vi "Main.vi"(10 "SerialPort":u8=1, 11 "Module Admin":refnum<class "Delacor_lib_QMH_Module Admin.lvclass">) -> ()   [LabVIEW 2020, in "SMC100.lvlib"]
doc: "This template is based off of the Queued Message Handler design pattern and the Queued Message Handler project template that ships with LabVIEW.\n\nThe main difference is that the queue is private to this module and communication between modules is performed via Broadcast and Request events.\n\nRequest events are wrapped in public API methods and are handled in the Event Handling Loop (EHL) of this VI. Any module can register for Broadcast events sent by this module. The EHL generates messages based on user interface actions.\n\nThe Message Handling Loop (MHL) processes messages generated by the EHL, or by other messages. The messages are string values, so new messages can be added easily to the Message Cases case structure in the MHL. Each message cluster can also provide an optional value for Message Data, which is a variant that can be converted to whatever message-specific data is required.\n_____\nBased on Delacor QMH Project Template 5.0.0.82."
uses:
  SMC100.lvlib
  <vilib>/Delacor/Delacor QMH/Libraries/Module Admin_class/Delacor_lib_QMH_Module Admin.lvclass
  Module Data--cluster.ctl
  Stop Argument--cluster.ctl
  <vilib>/Delacor/Delacor QMH/Libraries/Message Queue_class/Delacor_lib_QMH_Message Queue.lvclass/Delacor_lib_QMH_Message Queue.ctl
  <vilib>/Delacor/Delacor QMH/Libraries/Module Admin_class/Delacor_lib_QMH_Module Admin.lvclass/Delacor_lib_QMH_Module Admin.ctl
  Get Abs Position Argument--cluster.ctl
  Get Abs Position (Reply Payload)--cluster.ctl
  Set Abs Position Argument--cluster.ctl
  Move Home Argument--cluster.ctl
  <vilib>/Utility/miscctls.llb/LVPointTypeDef.ctl
  <vilib>/Delacor/Delacor QMH/Libraries/Message Queue_class/Delacor_lib_QMH_Enqueue Message (Single).vi
  <vilib>/Delacor/Delacor QMH/Libraries/Module Admin_class/Delacor_lib_QMH_Get External Launch.vi
  SMC100-Controller-Drivers/SMC100.llb/enter / leave disable state.vi
  <vilib>/Utility/error.llb/Error Cluster From Error Code.vi
  <vilib>/ErrorRing/Error Ring.xnode
  <vilib>/Delacor/Delacor QMH/Libraries/Message Queue_class/Delacor_lib_QMH_Message Queue.lvclass
panel:
  in  "Target Position":dbl format="%_4g"
  out "Absolute Position":dbl format="%_4g"
  out "Controller's state":string
  out "Controller's error":string
  out "error out":errorcluster
  out "Status":string
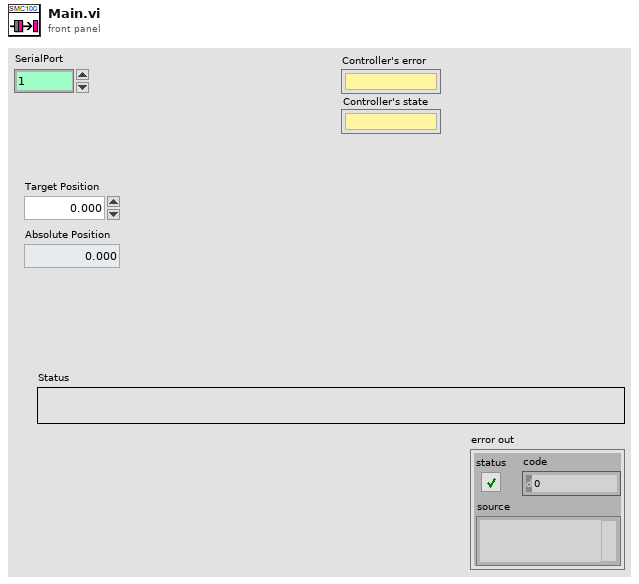
[diagram p1: front panel]
types:
  T1 = typedef "SMC100.lvlib/Request Events--cluster.ctl" = cluster{"Stop Module":refnum<user-event>, "Show Panel":refnum<user-event>, "Hide Panel":refnum<user-event>, "Get Module Execution Status":refnum<user-event>, "Show Diagram":refnum<user-event>, "Get Abs Position":refnum<user-event>, "Set Abs Position":refnum<user-event>, "Move Home":refnum<user-event>}
  T2 = typedef "SMC100.lvlib/Module Data--cluster.ctl" = cluster{"Status":string, "Visa Handle":refnum<visa-resource-name>}
  T3 = enum32{"invalid lock state", "Not Locked", "Locked (No Password)", "Password-protected"}
  T4 = typedef "SMC100.lvlib/Stop Argument--cluster.ctl" = cluster{"Origin":string, "Exit via Stop Module Req?":bool, "Wait for Module to stop?":bool}
  T5 = typedef "SMC100.lvlib/Get Abs Position Argument--cluster.ctl" = cluster{"Wait Notifier":refnum<notifier>, "wait for reply":bool}
  T6 = typedef "SMC100.lvlib/Set Abs Position Argument--cluster.ctl" = cluster{"Abolute Position":dbl}
  T7 = typedef "SMC100.lvlib/Move Home Argument--cluster.ctl" = cluster{"Boolean":bool}
  T8 = typedef "LVPointTypeDef.ctl" = cluster{"Horizontal":i16, "Vertical":i16}
  T9 = enum32{"Invalid", "Standard", "Closed", "Hidden", "Minimized", "Maximized"}
  T10 = typedef "SMC100.lvlib/Get Abs Position (Reply Payload)--cluster.ctl" = cluster{"Absolute Position":dbl, "Get Abs Position_error":errorcluster}
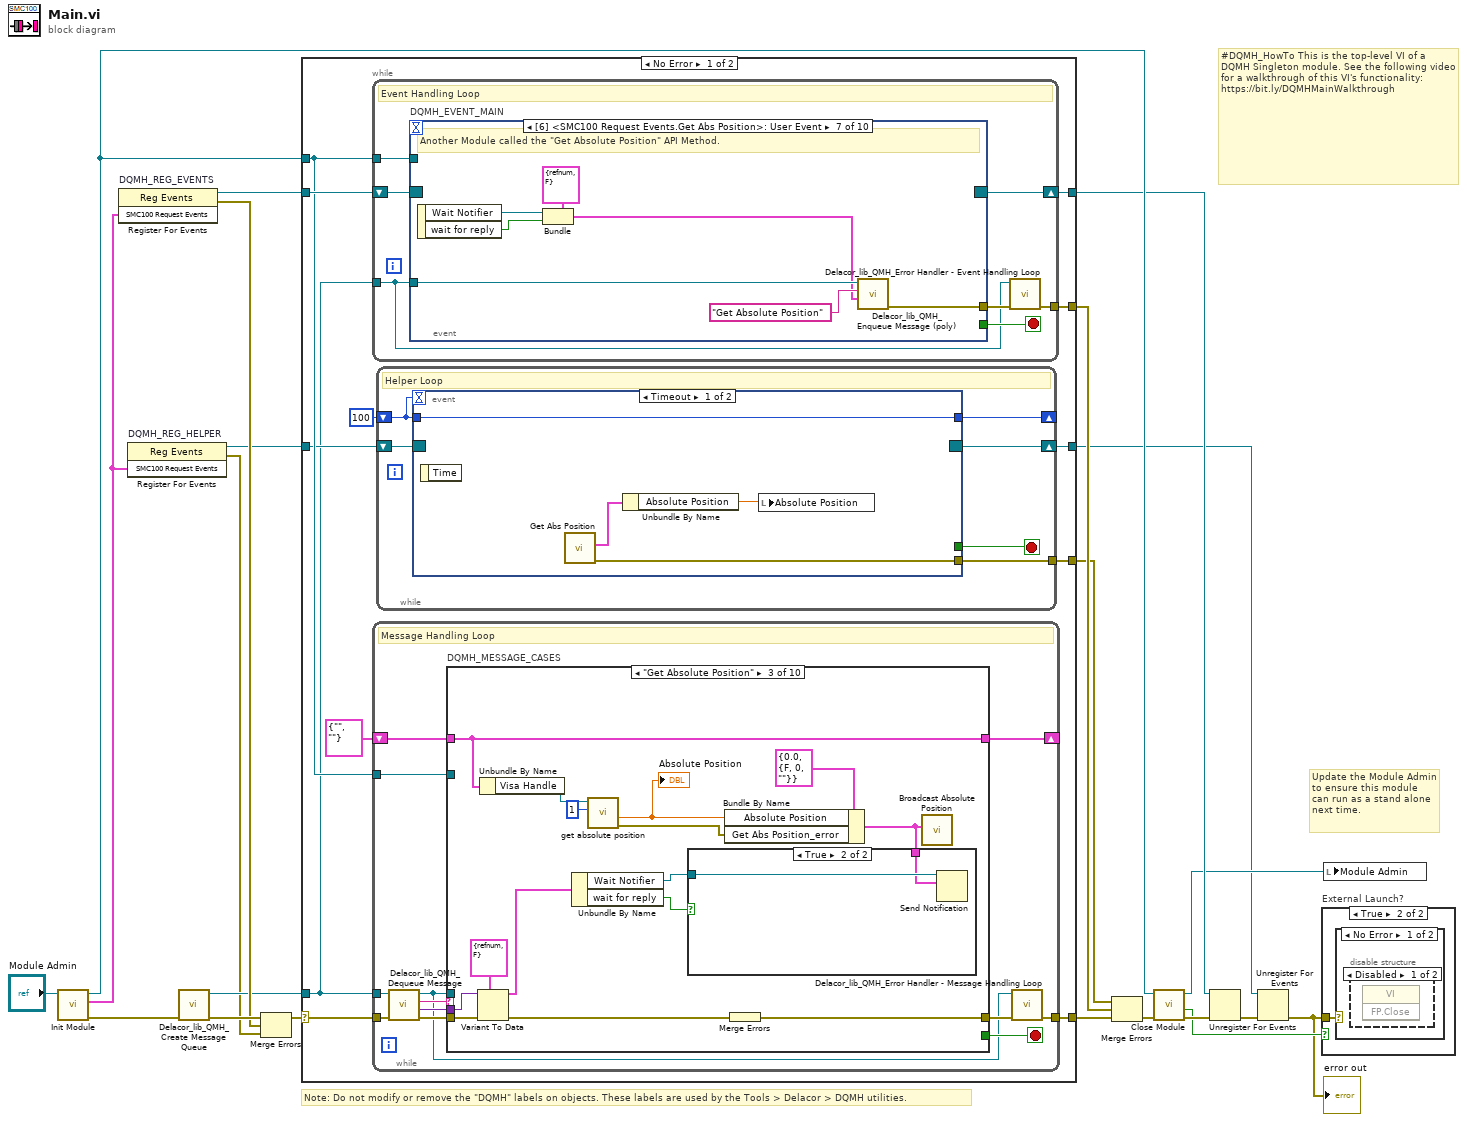
[diagram p0: block diagram]
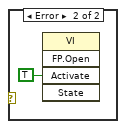
[diagram p4: hidden frame]
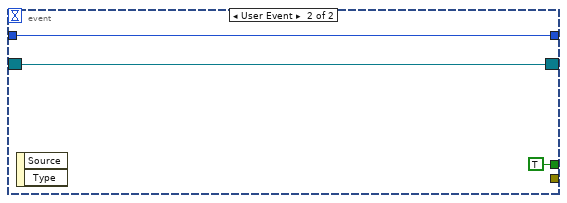
[diagram p5: hidden frame]
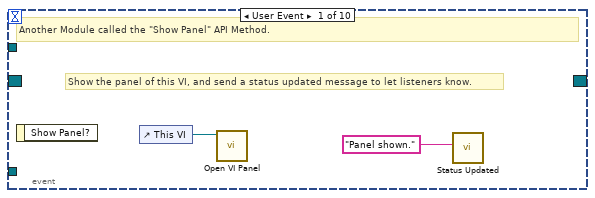
[diagram p6: hidden frame]
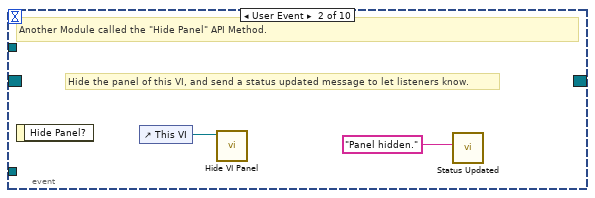
[diagram p7: hidden frame]
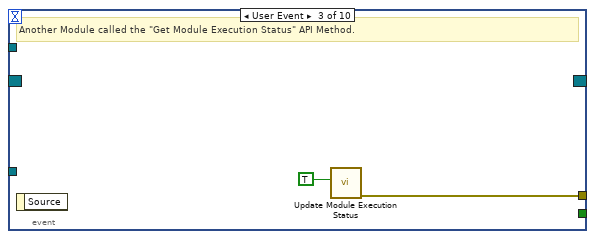
[diagram p8: hidden frame]
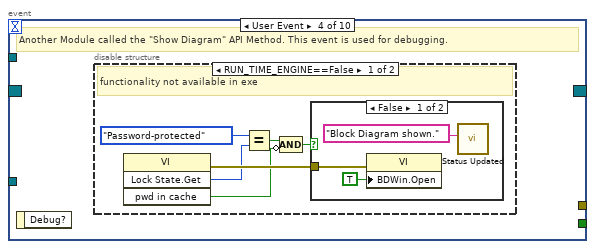
[diagram p9: hidden frame]
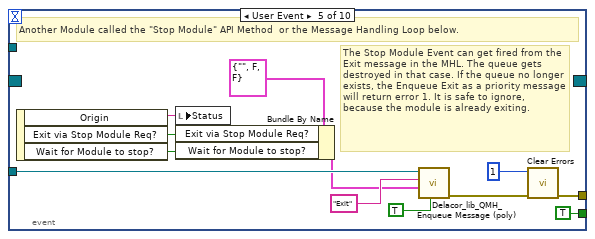
[diagram p12: hidden frame]
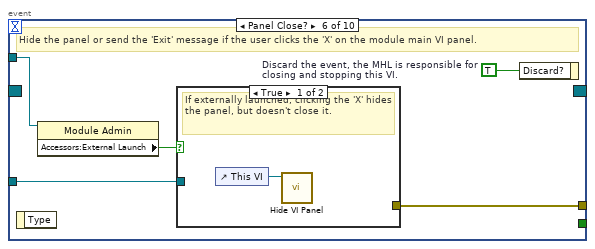
[diagram p13: hidden frame]
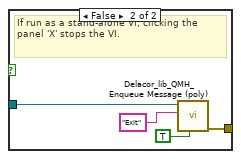
[diagram p14: hidden frame]
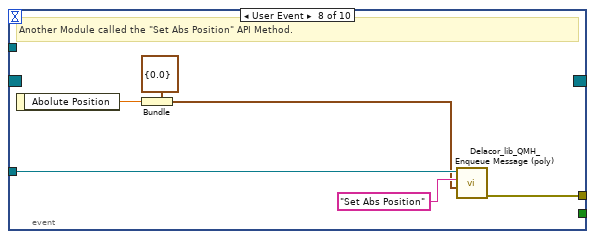
[diagram p15: hidden frame]
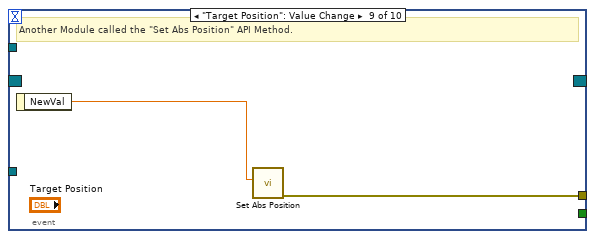
[diagram p16: hidden frame]
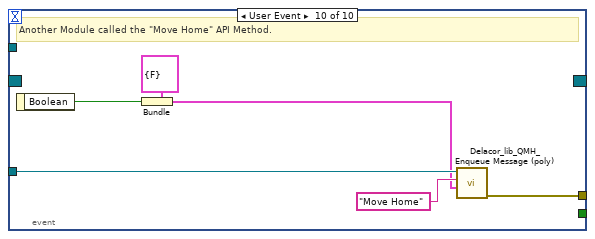
[diagram p17: hidden frame]
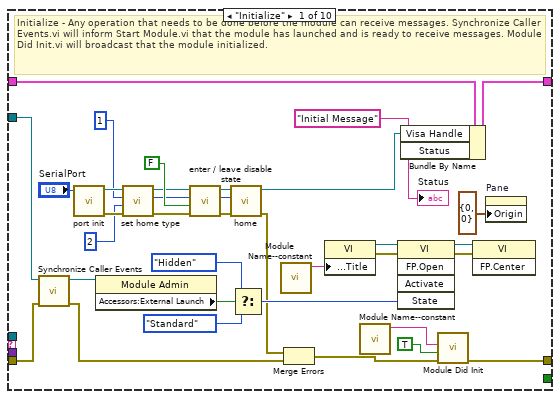
[diagram p18: hidden frame]
diagram:
  # "#DQMH_HowTo This is the top-level VI of a DQMH Singleton module. See the following video for a walkthrough of this VI's functionality: https://bit.ly/DQMHMainWalkthrough"
  # "Note: Do not modify or remove the \"DQMH\" labels on objects. These labels are used by the Tools > Delacor > DQMH utilities."
  # "Update the Module Admin to ensure this module can run as a stand alone next time."
  n1 = call "Init Module.vi"("Singleton Module Admin in"="Module Admin") -> ("error out"=w21:errorcluster, "SMC100 Request Events"=w4:T1, "Singleton Module Admin out"=w13:refnum<class "Delacor_lib_QMH_Module Admin.lvclass">)  [unwired: 8 in]
  n2 = register-events "DQMH_REG_EVENTS"(w4) -> (reference out=w11:refnum<event-registration>, error out=w14:errorcluster)  [unwired: 2 in]
  n3 = register-events "DQMH_REG_HELPER"(w4) -> (reference out=w6:refnum<event-registration>, error out=w5:errorcluster)  [unwired: 2 in]
  n4 = call <vilib>:"Delacor_lib_QMH_Create Message Queue.vi"("error in (no error)"=w21) -> ("error out"=w16:errorcluster, "Message Queue"=w10:refnum<class "Delacor_lib_QMH_Message Queue.lvclass">)  [unwired: 9 in]
  n5 = Merge Errors(w16, w14, w5) -> (w15:errorcluster)
  n6 = case shown="No Error" w15 {
    selector: w15 -> [w32 w260]
    tunnel: [w34 w259] -> w22
    tunnel: [w31 w265] -> w12
    tunnel: w11 -> [w29 w265]
    tunnel: w10 -> [w25 w258]
    tunnel: [w33 _] -> w19
    tunnel: w13 -> [w28 w261]
    tunnel: w6 -> [w26 w257]
    tunnel: [w24 w257] -> w2
    tunnel: [w23 _] -> w1
    frame No Error {
      n7 = while {
        tunnel: w25 -> [w48]
        shift-right: [w51] -> w31
        shift-left: w29 -> [w52]
        tunnel: [w53] -> w33
        tunnel: w28 -> [w49]
        stop <- w50 stop-if-true
        # "Event Handling Loop"
        n8 = event "DQMH_EVENT_MAIN" shown="[6] <SMC100 Request Events.Get Abs Position>: User Event" {
          selector: w52 -> [_ _ _ _ _ _ _ _ _ _]
          dyn-events: [_ _ _ _ _ _ _ _ _ _] -> w51
          timeout: _ -> [_ _ _ _ _ _ _ _ _ _]
          tunnel: [_ _ _ _ TRUE ("Discard?") _ _ _ _ _] -> w50
          tunnel: w48 -> [_ _ _ _ w77 w84 w98 w104 _ w112]
          tunnel: [_ _ w60 _ w80 w86 w92 w99 w106 w107] -> w54
          tunnel: w49 -> [_ _ _ _ _ w83 _ _ _ _]
          event User Event {
            # "Show the panel of this VI, and send a status updated message to let listeners know."
            # "Another Module called the \"Show Panel\" API Method."
            n9 = event-data() -> ()  [unwired: 1 in, 1 out]
            n10 = control-ref of="This VI"() -> (w56:refnum<vi>)
            n11 = call "Open VI Panel.vi"("VI"=w56) -> ()  [unwired: 10 in, 1 out]
            n12 = call "Status Updated.vi"("Status"="Panel shown." ("format string")) -> ()  [unwired: 10 in, 1 out]
          }
          event User Event {
            # "Hide the panel of this VI, and send a status updated message to let listeners know."
            # "Another Module called the \"Hide Panel\" API Method."
            n13 = event-data() -> ()  [unwired: 1 in, 1 out]
            n14 = control-ref of="This VI"() -> (w58:refnum<vi>)
            n15 = call "Hide VI Panel.vi"("VI"=w58) -> ()  [unwired: 10 in, 1 out]
            n16 = call "Status Updated.vi"("Status"="Panel hidden." ("format string")) -> ()  [unwired: 10 in, 1 out]
          }
          event User Event {
            # "Another Module called the \"Get Module Execution Status\" API Method."
            n17 = event-data() -> ()  [unwired: 1 in, 1 out]
            n18 = call "Update Module Execution Status.vi"("Running?"=TRUE) -> ("error out"=w60:errorcluster)  [unwired: 10 in]
          }
          event User Event {
            # "Another Module called the \"Show Diagram\" API Method. This event is used for debugging."
            n19 = event-data() -> ()  [unwired: 1 in, 1 out]
            n20 = disable-structure shown="RUN_TIME_ENGINE==False" {
              frame condition #0 (active) {
                # "functionality not available in exe"
                n21 = invoke class="VI" method="Lock State.Get"() -> (error out=w66:errorcluster, "Get Lock State"=w65:T3, "pwd in cache"=w62:bool)  [unwired: 4 in, 1 out]
                n22 = Equal?(x=T3."Password-protected", y=w65) -> (x = y?=w63:bool)
                n23 = Compound Arithmetic op=AND(w63, invert w62) -> (w61:bool)
                n24 = case shown="False" w61 {
                  tunnel: w66 -> [w69 _]
                  frame False {
                    n25 = property class="VI"(error in=w69, "BDWin.Open"=TRUE ("Block Diagram Window:Open")) -> ()  [unwired: 1 in, 2 out]
                    n26 = call "Status Updated.vi"("Status"="Block Diagram shown." ("format string")) -> ()  [unwired: 10 in, 1 out]
                  }
                  frame True {
                    # "Password-protected VI, and the password is not in the cache. Do not show the diagram."
                  }
                }
              }
              frame condition #1 {
              }
            }
          }
          event User Event {
            # "The Stop Module Event can get fired from the Exit message in the MHL. The queue gets destroyed in that case. If the queue no longer exists, the Enqueue Exit as a priority message will return error 1. It is safe to ignore, because the module is already exiting."
            # "Another Module called the \"Stop Module\" API Method  or the Message Handling Loop below."
            n27 = event-data() -> ("Origin"=w76:string, "Exit via Stop Module Req?"=w72:bool, "Wait for Module to stop?"=w71:bool)  [unwired: 1 in]
            n28 = local write "Status"(w76) -> ()
            n29 = Bundle By Name(cluster=T4 {"Origin"="", "Exit via Stop Module Req?"=FALSE, "Wait for Module to stop?"=FALSE} ("Stop Argument"), "Exit via Stop Module Req?"=w72, "Wait for Module to stop?"=w71) -> (w70:T4)
            n30 = call-poly <vilib>:"Delacor_lib_QMH_Enqueue Message (poly).vi"("Priority Message? (F)"=TRUE, "Message Data"=w70, "Message"="Exit", "Message Queue in"=w77) -> ("error out"=w81:errorcluster)  [unwired: 6 in, 1 out]
            n31 = call <vilib>:"Clear Errors.vi"("error in (no error)"=w81, "specific error code to clear (0: all)"=1) -> ("error out"=w80:errorcluster)  [unwired: 4 in, 1 out]
          }
          event Panel Close? {
            w85 = TRUE  # Discard the event, the MHL is responsible for closing and stopping this VI.
            # "Hide the panel or send the 'Exit' message if the user clicks the 'X' on the module main VI panel."
            n32 = event-data() -> ()  [unwired: 1 in, 1 out]
            n33 = property class="Module Admin"(reference=w83) -> ("Accessors:External Launch"=w82:bool)  [unwired: 1 in, 2 out]
            n34 = case shown="True" w82 {
              tunnel: w84 -> [_ w90]
              tunnel: [_ w91] -> w86
              frame True {
                # "If externally launched, clicking the 'X' hides the panel, but doesn't close it."
                n35 = control-ref of="This VI"() -> (w87:refnum<vi>)
                n36 = call "Hide VI Panel.vi"("VI"=w87) -> ()  [unwired: 10 in, 1 out]
              }
              frame False {
                # "If run as a stand-alone VI, clicking the panel 'X' stops the VI."
                n37 = call-poly <vilib>:"Delacor_lib_QMH_Enqueue Message (poly).vi"("Priority Message? (F)"=TRUE, "Message"="Exit", "Message Queue in"=w90) -> ("error out"=w91:errorcluster)  [unwired: 7 in, 1 out]
              }
            }
            n38 = event-data("Discard?"=w85) -> ()  [unwired: 1 in, 1 out]
          }
          event User Event {
            # "Another Module called the \"Get Absolute Position\" API Method."
            n39 = event-data() -> ("Wait Notifier"=w94:refnum<notifier>, "wait for reply"=w93:bool)  [unwired: 1 in]
            n40 = Bundle(cluster=T5 {"Wait Notifier"=refnum, "wait for reply"=FALSE} ("Get Absolute Position Argument"), "Wait Notifier"=w94, "wait for reply"=w93) -> (w95:T5)
            n41 = call-poly <vilib>:"Delacor_lib_QMH_Enqueue Message (poly).vi"("Message Data"=w95, "Message"="Get Absolute Position", "Message Queue in"=w98) -> ("error out"=w92:errorcluster)  [unwired: 7 in, 1 out]
          }
          event User Event {
            # "Another Module called the \"Set Abs Position\" API Method."
            n42 = event-data() -> ("Abolute Position"=w100:dbl)  [unwired: 1 in]
            n43 = Bundle(cluster=T6 {"Abolute Position"=0.0} ("Set Abs Position Argument"), "Abolute Position"=w100) -> (w101:T6)
            n44 = call-poly <vilib>:"Delacor_lib_QMH_Enqueue Message (poly).vi"("Message Data"=w101, "Message"="Set Abs Position", "Message Queue in"=w104) -> ("error out"=w99:errorcluster)  [unwired: 7 in, 1 out]
          }
          event "Target Position": Value Change {
            # "Another Module called the \"Set Abs Position\" API Method."
            n45 = event-data() -> ("NewVal"=w105:dbl)  [unwired: 1 in]
            n46 = call "Set Abs Position.vi"("Abolute Position"=w105) -> ("error out"=w106:errorcluster)  [unwired: 10 in]
          }
          event User Event {
            # "Another Module called the \"Move Home\" API Method."
            n47 = event-data() -> ("Boolean"=w108:bool)  [unwired: 1 in]
            n48 = Bundle(cluster=T7 {"Boolean"=FALSE} ("Move Home Argument"), "Boolean"=w108) -> (w109:T7)
            n49 = call-poly <vilib>:"Delacor_lib_QMH_Enqueue Message (poly).vi"("Message Data"=w109, "Message"="Move Home", "Message Queue in"=w112) -> ("error out"=w107:errorcluster)  [unwired: 7 in, 1 out]
          }
        }
        n50 = call-dynamic "Delacor_lib_QMH_Error Handler - Event Handling Loop.vi"("error in (no error)"=w54, "Message Queue in"=w48) -> ("dup error in"=w53:errorcluster)  [unwired: 8 in, 1 out]
      }
      n51 = while {
        tunnel: w25 -> [w115]
        shift-right: [w119] -> _
        shift-left: T2 {"Status"="", "Visa Handle"=""} ("Data Cluster") -> [w120]
        tunnel: w32 -> [w123]
        tunnel: [w121] -> w34
        tunnel: w28 -> [w113]
        stop <- w118 stop-if-true
        # "Message Handling Loop"
        n52 = call-dynamic "Delacor_lib_QMH_Dequeue Message.vi"("error in (no error)"=w123, "Message Queue in"=w115) -> ("error out"=w122:errorcluster, "Message Data"=w116:variant, "Message"=w117:string, "Message Queue out"=w114:refnum<class "Delacor_lib_QMH_Message Queue.lvclass">)  [unwired: 6 in]
        n53 = case "DQMH_MESSAGE_CASES" shown="\"Get Absolute Position\"" w117 {
          selector: w117 -> [_ _ _ _ _ _ _ _ _ w244]
          tunnel: w114 -> [_ _ _ _ _ _ _ w210 w236 _]
          tunnel: w122 -> [w157 w161 w176 w188 w201 w204 w206 w217 w242 w246]
          tunnel: [w155 w161 w167 w180 w193 w203 w206 w213 w239 w247] -> w124
          tunnel: w120 -> [w146 w160 w166 w184 w195 w202 w205 w212 w227 w245]
          tunnel: [w145 w160 w166 w184 w195 w202 w205 w212 w227 w245] -> w119
          tunnel: [_ _ _ _ _ _ _ _ w235 _] -> w118
          tunnel: w116 -> [_ _ w174 w187 w199 _ _ w211 w234 _]
          tunnel: w113 -> [w147 _ _ _ _ _ _ w209 w229 _]
          frame "Initialize" {
            w140 = "Initial Message" ("Initial Message")
            # "Initialize - Any operation that needs to be done before the module can receive messages. Synchronize Caller Events.vi will inform Start Module.vi that the module has launched and is ready to receive messages. Module Did Init.vi will broadcast that the module initialized."
            n54 = call "Synchronize Caller Events.vi"("error in (no error)"=w157, "Singleton Module Admin in"=w147) -> ("error out"=w156:errorcluster, "Singleton Module Admin out"=w142:refnum<class "Delacor_lib_QMH_Module Admin.lvclass">)  [unwired: 8 in]
            n55 = call "port init.vi"("SerialPort"="SerialPort") -> ("error out"=w132:errorcluster, "Visa Handle"=w130:refnum<visa-resource-name>)  [unwired: 3 in]
            n56 = property class="Module Admin"(reference=w142) -> ("Accessors:External Launch"=w151:bool)  [unwired: 1 in, 2 out]
            n57 = call "set home type.vi"("error in"=w132, "Home type value :\n0 use MZ switch and encoder Index\n1 use current position as HOME\n2 use MZ switch only\n3 use EoR- switch and encoder Index\n4 use EoR- switch only"=2 ("Home type value :\n0 use MZ switch and encoder Index\n1 use current position as HOME\n2 use MZ switch only\n3 use EoR- switch and encoder Index\n4 use EoR- switch only"), "Axis in"=1, "VISA Handle in"=w130) -> ("error out"=w131:errorcluster, "Axis out"=w126:i32, "VISA Handle out"=w127:refnum<visa-resource-name>)  [unwired: 2 in, 1 out]
            n58 = call "enter / leave disable state.vi"("error in"=w131, "enter disable state (True)"=FALSE, "Axis in"=w126, "VISA handle in"=w127) -> ("error out"=w135:errorcluster, "Axis out"=w125:i32, "VISA handle out"=w134:refnum<visa-resource-name>)  [unwired: 4 in, 1 out]
            n59 = call "home.vi"("error in"=w135, "Axis in"=w125, "VISA Handle in"=w134) -> ("error out"=w137:errorcluster, "VISA Handle out"=w136:refnum<visa-resource-name>)  [unwired: 3 in, 2 out]
            n60 = Select(t=T9."Hidden" ("State"), s=w151, f=T9."Standard" ("State")) -> (s? t:f=w148:T9)
            n61 = call "Module Name--constant.vi"() -> ("Module Name"=w154:string)  [unwired: 11 in]
            n62 = Merge Errors(w137, w156) -> (w138:errorcluster)
            n63 = property class="VI"("Front Panel.Title"=w154) -> (reference out=w153:refnum<vi>, error out=w159:errorcluster)  [unwired: 2 in]
            n64 = call "Module Name--constant.vi"() -> ("Module Name"=w143:string)  [unwired: 11 in]
            n65 = invoke class="VI" method="FP.Open"(reference=w153, error in=w159, "State"=w148) -> (reference out=w152:refnum<vi>, error out=w158:errorcluster)  [unwired: 2 in, 3 out]
            n66 = Bundle By Name(cluster=w146, "Visa Handle"=w136, "Status"=w140) -> (w145:T2)
            n67 = call "Module Did Init.vi"("error in (no error)"=w138, "Initialized?"=TRUE, "Origin"=w143) -> ("error out"=w155:errorcluster)  [unwired: 8 in]
            n68 = invoke class="VI" method="FP.Center"(reference=w152, error in=w158) -> ()  [unwired: 1 in, 3 out]
            n69 = property on="Pane" class="Pane"("Origin"=T8 {"Horizontal"=0, "Vertical"=0}) -> ()  [unwired: 2 in, 2 out]
            "Status" <- w140
          }
          frame "--- Module Specific ---" {
            # "Separator -- The following cases handle messages specific to this Module."
          }
          frame "Get Absolute Position" {
            n70 = Variant To Data(error in=w176, type=T5 {"Wait Notifier"=refnum, "wait for reply"=FALSE} ("Get Absolute Position Argument"), Variant=w174) -> (data=w172:T5, error out=w175:errorcluster)
            n71 = Unbundle By Name(w166) -> ("Visa Handle"=w165:refnum<visa-resource-name>)
            n72 = Unbundle By Name(w172) -> ("Wait Notifier"=w171:refnum<notifier>, "wait for reply"=w170:bool)
            n73 = call "get absolute position.vi"("Axis in"=1, "VISA Handle in"=w165) -> ("error out"=w164:errorcluster, "Target position (units)"=w162:dbl)  [unwired: 3 in, 3 out]
            "Absolute Position" <- w162
            n74 = Bundle By Name(cluster=T10 {"Absolute Position"=0.0, "Get Abs Position_error"={"status"=FALSE, "code"=0, "source"=""}} ("Get Absolute Position (Reply Payload)"), "Absolute Position"=w162, "Get Abs Position_error"=w164) -> (w169:T10)
            n75 = case shown="True" w170 {
              tunnel: w171 -> [_ w178]
              tunnel: w169 -> [_ w177]
              frame False {
              }
              frame True {
                n76 = Send Notification(notification=w177, notifier=w178) -> ()  [unwired: 1 in, 2 out]
              }
            }
            n77 = Merge Errors(w175) -> (w167:errorcluster)
            n78 = call "Broadcast Absolute Position.vi"("Reply Payload"=w169) -> ()  [unwired: 10 in, 1 out]
          }
          frame "Set Abs Position" {
            n79 = Variant To Data(error in=w188, type=T6 {"Abolute Position"=0.0} ("Set Abs Position Argument"), Variant=w187) -> (data=w185:T6, error out=w181:errorcluster)
            n80 = Unbundle By Name(w184) -> ("Visa Handle"=w183:refnum<visa-resource-name>)
            n81 = Unbundle By Name(w185) -> ("Abolute Position"=w182:dbl)
            n82 = call "Move absolute.vi"("error in"=w181, "New target position (units)"=w182, "Axis in"=1, "VISA Handle in"=w183) -> ("error out"=w180:errorcluster)  [unwired: 2 in, 3 out]
          }
          frame "Move Home" {
            w189 = 1 ("Axis in")
            n83 = Variant To Data(error in=w201, type=T7 {"Boolean"=FALSE} ("Move Home Argument"), Variant=w199) -> (data=w197:T7, error out=w200:errorcluster)
            n84 = Unbundle By Name(w195) -> ("Visa Handle"=w194:refnum<visa-resource-name>)
            n85 = Unbundle By Name(w197) -> ()  [unwired: 1 out]
            n86 = call "home.vi"("error in"=w200, "Axis in"=w189, "VISA Handle in"=w194) -> ("error out"=w196:errorcluster, "VISA Handle out"=w192:refnum<visa-resource-name>)  [unwired: 3 in, 2 out]
            n87 = call "tell controller status.vi"("VISA Handle in"=w192, "Axis in"=w189, "error in"=w196) -> ("Controller's error"=→"Controller's error":string, "Controller's state"=→"Controller's state":string, "error out"=w193:errorcluster)  [unwired: 7 in, 3 out]
          }
          frame "---Copy This Frame---" {
            # "Duplicate this frame when creating new messages.  Change this comment in the duplicated frame to describe this message."
            n88 = Merge Errors(w204) -> (w203:errorcluster)
          }
          frame "--- Exit and Error Handling---" {
            # "Separator - The following cases handle errors and exit messages."
          }
          frame "Error" {
            # "#CodeRecommended - If you ever change the name of this \"Error\" message, you'll need to update the name in the Check Loop Error.vi as well."
            # "#CodeRecommended - If the module is running in standalone mode (External Launch = FALSE), this code will pop up an error dialog and call the 'Exit' message if an error occurs. Add more fine-grained error handling here."
            # "Error - Check the error message data and respond accordingly. This message is sent by the \"Error Handler\" VIs at the end of each loop in this application."
            n89 = property class="Module Admin"(reference=w209) -> ("Accessors:External Launch"=w208:bool)  [unwired: 1 in, 2 out]
            n90 = Variant To Data(error in=w217, type=errorcluster {"status"=FALSE, "code"=0, "source"=""} ("error constant"), Variant=w211) -> (data=w218:errorcluster, error out=w215:errorcluster)
            n91 = call "Module Name--constant.vi"() -> ("Module Name"=w207:string)  [unwired: 11 in]
            n92 = call "Error Reported.vi"("Additional Information"=w207, "Error"=w218) -> ()  [unwired: 9 in, 1 out]
            n93 = case shown="False" w208 {
              tunnel: [w223 _] -> w214
              tunnel: w210 -> [w221 _]
              tunnel: w218 -> [w222 _]
              frame False {
                # "If the module is running standalone, then pop up an error dialog and call the \"Exit\" message."
                n94 = call <vilib>:"Simple Error Handler.vi"("error in (no error)"=w222) -> ()  [unwired: 4 in, 5 out]
                n95 = call-poly <vilib>:"Delacor_lib_QMH_Enqueue Message (poly).vi"("Priority Message? (F)"=TRUE, "Message"="Exit", "Message Queue in"=w221) -> ("error out"=w223:errorcluster)  [unwired: 7 in, 1 out]
              }
              frame True {
                # "If the module was launched externally, calling the Error Reported broadcast VI is the only action performed by the \"Error\" message. The module's caller can then process the error appropriately."
              }
            }
            n96 = Merge Errors(w215, w214) -> (w213:errorcluster)
            n97 = local write "error out"(w213) -> ()
          }
          frame "Exit" {
            w233 = 91  # 91: not all Exit messages will have an argument
            w235 = TRUE  # Stop the VI
            # "Release the message queue reference"
            # "Exit - Exit the application."
            n98 = control-ref of="This VI"() -> (w230:refnum<vi>)
            n99 = Variant To Data(error in=w242, type=T4 {"Origin"="", "Exit via Stop Module Req?"=FALSE, "Wait for Module to stop?"=FALSE} ("Stop Argument"), Variant=w234) -> (data=w231:T4, error out=w238:errorcluster)
            n100 = call "Handle Exit.vi"("Stop Argument"=w231, "Admin in"=w229, "VI reference"=w230) -> ("error out"=w237:errorcluster)  [unwired: 7 in, 1 out]
            n101 = call <vilib>:"Clear Errors.vi"("error in (no error)"=w238, "specific error code to clear (0: all)"=w233) -> ("error out"=w241:errorcluster)  [unwired: 4 in, 1 out]
            n102 = Unbundle By Name(w227) -> ("Visa Handle"=w225:refnum<visa-resource-name>)
            n103 = call "enter / leave disable state.vi"("error in"=w237, "VISA handle in"=w225) -> ("error out"=w226:errorcluster, "VISA handle out"=w224:refnum<visa-resource-name>)  [unwired: 6 in, 2 out]
            n104 = call-dynamic "Delacor_lib_QMH_Release Message Queue.vi"("error in (no error)"=w241, "Message Queue"=w236) -> ("error out"=w240:errorcluster)  [unwired: 9 in]
            n105 = VISA Close(VISA resource name=w224, error in (no error)=w226) -> (error out=w228:errorcluster)
            n106 = Merge Errors(w240, w228) -> (w239:errorcluster)
          }
          frame Default {
            # "'Default' case only runs if there is a message that isn't defined in any of the other cases.  Output a programming error."
            n107 = call "Module Name--constant.vi"() -> ("Module Name"=w243:string)  [unwired: 11 in]
            n108 = xnode "Error Ring"("parameter 0"=w244, "parameter 1"=w243) -> ("error out"=w248:errorcluster)
            n109 = Merge Errors(w246, w248) -> (w247:errorcluster)
          }
        }
        n110 = call-dynamic "Delacor_lib_QMH_Error Handler - Message Handling Loop.vi"("error in (no error)"=w124, "Message Queue in"=w114) -> ("dup error in"=w121:errorcluster)  [unwired: 8 in, 1 out]
      }
      n111 = while {
        shift-right: [w37] -> _
        shift-left: 100 -> [w40]
        shift-right: [w36] -> w24
        shift-left: w26 -> [w39]
        tunnel: [w35] -> w23
        stop <- w38 stop-if-true
        # "Helper Loop"
        n112 = event shown="[0] Timeout" {
          selector: w39 -> [_ w46]
          dyn-events: [_ w46] -> w36
          timeout: w40 -> [_ _]
          tunnel: w40 -> [w44 w45]
          tunnel: [_ TRUE] -> w38
          tunnel: [w44 w45] -> w37
          tunnel: [w43 _] -> w35
          event Timeout {
            n113 = event-data() -> ()  [unwired: 1 in, 1 out]
            n114 = call "Get Abs Position.vi"() -> ("error out"=w43:errorcluster, "Reply Payload"=w42:T10)  [unwired: 9 in, 1 out]
            n115 = Unbundle By Name(w42) -> ("Absolute Position"=w41:dbl)
            n116 = local write "Absolute Position"(w41) -> ()
          }
          event User Event {
            n117 = event-data() -> ()  [unwired: 1 in, 2 out]
          }
        }
      }
    }
    frame Error {
      # "Synchronize Caller Events.vi will inform Start Module.vi that the module has launched and will let the code calling Start Module.vi register for broadcasts and would permit the caller receive the broadcast that an error occurred at launch time."
      n118 = call-dynamic "Delacor_lib_QMH_Release Message Queue.vi"("error in (no error)"=w260, "Message Queue"=w258) -> ("error out"=w259:errorcluster)  [unwired: 9 in]
      n119 = call "Synchronize Caller Events.vi"("Singleton Module Admin in"=w261) -> ("error out"=w266:errorcluster)  [unwired: 9 in, 1 out]
      n120 = call "Module Name--constant.vi"() -> ("Module Name"=w264:string)  [unwired: 11 in]
      n121 = Format Into String(format string="An error occurred during initialization. %s is no longer running.", w264) -> (resulting string=w262:string)  [unwired: 2 in, 1 out]
      n122 = Merge Errors(w259, w266) -> (w267:errorcluster)
      n123 = call "Error Reported.vi"("Additional Information"=w262, "Error"=w267) -> ()  [unwired: 9 in, 1 out]
    }
  }
  n124 = Merge Errors(w1, w19, w22) -> (w18:errorcluster)
  n125 = call "Close Module.vi"("error in (no error)"=w18, "Module Admin in"=w13) -> ("error out"=w20:errorcluster, "External Launch"=w7:bool, "Module Admin out"=w8:refnum<class "Delacor_lib_QMH_Module Admin.lvclass">)  [unwired: 7 in]
  n126 = Unregister For Events(event registration refnum=w12, error in=w20) -> (error out=w17:errorcluster)
  n127 = Unregister For Events(event registration refnum=w2, error in=w17) -> (error out=w3:errorcluster)
  "error out" <- w3
  n128 = case "External Launch?" shown="True" w7 {
    tunnel: w3 -> [_ w268]
    frame False {
    }
    frame True {
      n129 = case shown="No Error" w268 {
        frame No Error {
          n130 = disable-structure shown="Disabled" {
            frame Disabled {
              n131 = invoke class="VI" method="FP.Close"() -> ()  [unwired: 3 in, 3 out]
            }
            frame Enabled {
            }
          }
        }
        frame Error {
          n132 = invoke class="VI" method="FP.Open"("Activate"=TRUE ("Activate?")) -> ()  [unwired: 4 in, 5 out]
        }
      }
    }
  }
  n133 = local write "Module Admin"(w8) -> ()
